vi "Peak Detector (obs 2010).vi"(4 "end of data (T)":bool=TRUE, 6 "initialize (T)":bool=TRUE, 8 "peaks/valleys":enum32{"Peaks", "Valleys"}(ring), 9 "width":i32=3 min=3, 10 "threshold":dbl format="%0.2f", 11 "X":dbl[](array[numeric])) -> (0 "error":i32, 1 "2nd Derivatives":dbl[](array[numeric]), 2 "Amplitudes":dbl[](array[numeric]), 3 "Locations":dbl[](array[numeric]), 5 "# found":i32)   [LabVIEW 2017, in "NI_AALPro.lvlib"]
doc: "Finds the location, amplitude, and second derivative of peaks or valleys in the input signal."
uses:
  NI_AALPro.lvlib
  <resource>/lvanlys.dll
panel:
  # "This VI is obsolete !\nYou should replace this VI in your digram with the Peak Detector VI."
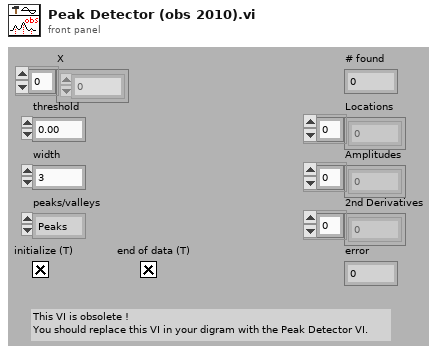
[diagram p1: front panel]
types:
  T1 = cluster{"Span":i32, "Index":i32, "NHistoryPts":i32, "Len":i32, "PrevSign":i32, "unused":i32, "RinvQt (pointer)":u32, "FitBuffer (pointer)":u32, "History (pointer)":u32, "PrevCoeff (pointer)":u32, "Data (pointer)":u32, "slack for RinvQt":u32, "slack for FitBuffer":u32, "slack for History":u32, "slack for PrevCoeff":u32, "slack for Data":u32}
  T2 = cluster{"X":dbl[], "threshold":dbl, "Span":i32, "peaks/valleys":enum32{"Peaks", "Valleys"}, "Array Constant":dbl[], "Array Constant":dbl[], "Array Constant":dbl[], i32, i32}
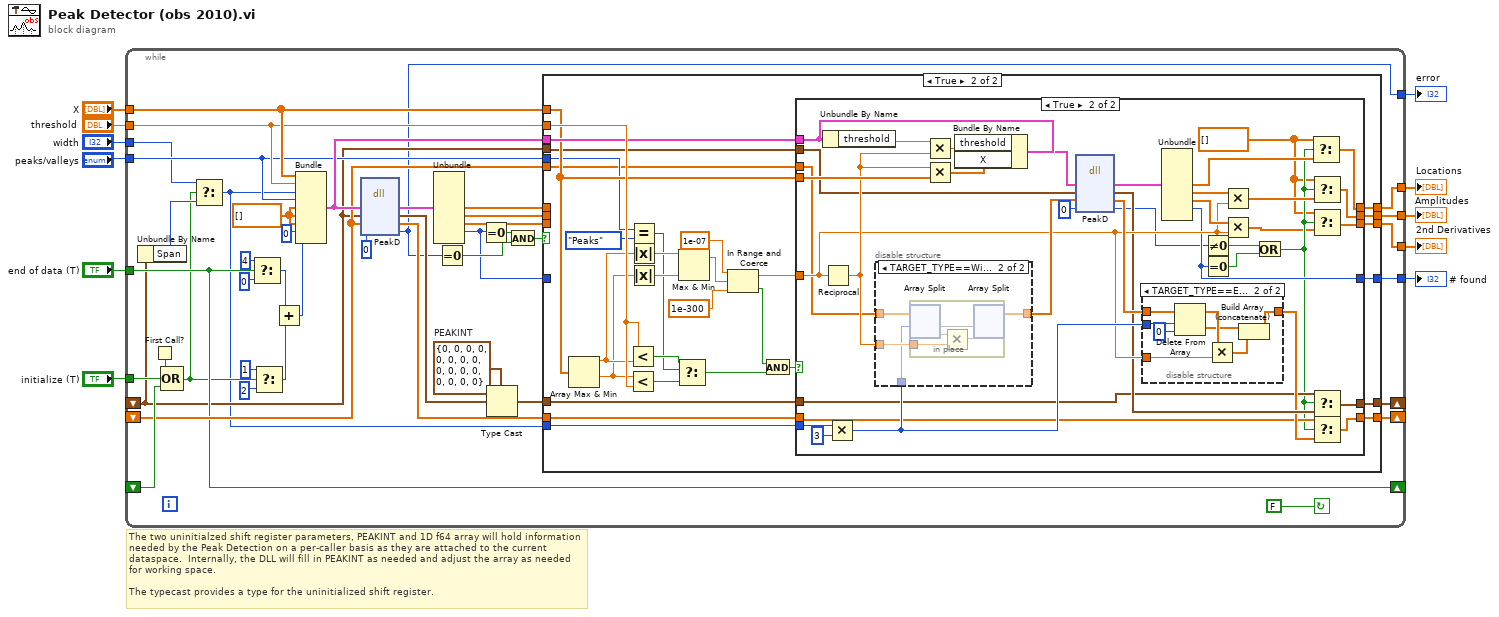
[diagram p0: block diagram]
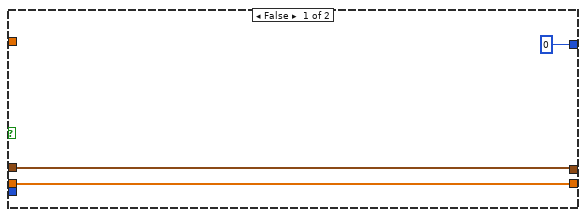
[diagram p3: hidden frame]
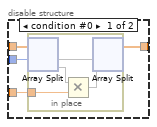
[diagram p4: hidden frame]
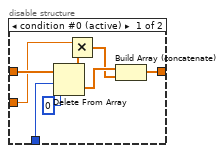
[diagram p5: hidden frame]
diagram:
  # "The two uninitialzed shift register parameters, PEAKINT and 1D f64 array will hold information needed by the Peak Detection on a per-caller basis as they are attached to the current dataspace.  Internally, the DLL will fill in PEAKINT as needed and adjust the array as needed for working space.\n\nThe typecast provides a type for the uninitialized shift register."
  n1 = while {
    shift-left: _ -> [w31]
    shift-right: [w33] -> _
    shift-left: _ -> [w17]
    shift-right: [w35] -> _
    shift-right: [w27] -> _
    shift-left: _ -> [w41]
    tunnel: "X" -> [w30]
    tunnel: "threshold" -> [w29]
    tunnel: "width" -> [w13]
    tunnel: "peaks/valleys" -> [w28]
    tunnel: "end of data (T)" -> [w27]
    tunnel: "initialize (T)" -> [w26]
    tunnel: [w12] -> w5
    tunnel: [w25] -> w4
    tunnel: [w24] -> w3
    tunnel: [w23] -> w2
    tunnel: [w22] -> w1
    stop <- FALSE continue-if-true
    w42 = T1 {"Span"=0, "Index"=0, "NHistoryPts"=0, "Len"=0, "PrevSign"=0, "unused"=0, "RinvQt (pointer)"=0, "FitBuffer (pointer)"=0, "History (pointer)"=0, "PrevCoeff (pointer)"=0, "Data (pointer)"=0, "slack for RinvQt"=0, "slack for FitBuffer"=0, "slack for History"=0, "slack for PrevCoeff"=0, "slack for Data"=0}  # PEAKINT
    w45 = dbl[] [] ("Array Constant")
    n2 = Unbundle By Name(w17) -> ("Span"=w16:i32)
    n3 = First Call?() -> (First Call?: T/F=w40:bool)
    n4 = Compound Arithmetic op=OR(w40, w26, w41) -> (w15:bool)
    n5 = Select(t=w13, s=w15, f=w16) -> (s? t:f=w14:i32)
    n6 = Select(t=4, s=w27, f=0) -> (s? t:f=w54:i32)
    n7 = Select(t=1, s=w15, f=2) -> (s? t:f=w55:i32)
    n8 = Add(x=w54, y=w55) -> (x+y=w48:i32)
    n9 = Bundle("X"=w30, "threshold"=w29, "Span"=w14, "peaks/valleys"=w28, "Array Constant"=w45, "Array Constant"=w45, "Array Constant"=w45, 0, w48) -> (w32:T2)  [unwired: 1 out]
    n10 = dll-call lib="C:/Program Files (x86)/National Instruments/LabVIEW 2017/resource/lvanlys.*" fn="PeakD"("PeakApp"=w32, "pPEAKINT"=w17, "SavedData"=w31, "pErr"=0) -> ("PeakApp"=w47:T2, "pPEAKINT"=w43:T1, "SavedData"=w34:dbl[], "pErr"=w12:i32)  [unwired: 3 in, 3 out]
    n11 = Unbundle(w47) -> ("Array Constant"=w37:dbl[], "Array Constant"=w38:dbl[], "Array Constant"=w39:dbl[], w18:i32)  [unwired: 5 out]
    n12 = Equal To 0?(x=w12) -> (x = 0?=w20:bool)
    n13 = Equal To 0?(x=w18) -> (x = 0?=w21:bool)
    n14 = Type Cast(type=w42, x=w43) -> (*(type *) &x=w36:T1)
    n15 = And(x=w21, y=w20) -> (x .and. y?=w19:bool)
    n16 = case shown="True" w19 {
      tunnel: w39 -> [w59 _]
      tunnel: w38 -> [w60 _]
      tunnel: w37 -> [w61 _]
      tunnel: w30 -> [_ w72]
      tunnel: w29 -> [_ w91]
      tunnel: w28 -> [_ w69]
      tunnel: w34 -> [w57 w80]
      tunnel: w36 -> [w58 w62]
      tunnel: [w58 w79] -> w35
      tunnel: [w57 w78] -> w33
      tunnel: [w59 w77] -> w23
      tunnel: [w60 w76] -> w24
      tunnel: [w61 w75] -> w25
      tunnel: w32 -> [_ w73]
      tunnel: w17 -> [_ w71]
      tunnel: w31 -> [_ w68]
      tunnel: [w56 w67] -> w22
      tunnel: w18 -> [w56 _]
      tunnel: w14 -> [_ w63]
      frame False {
      }
      frame True {
        n17 = Array Max & Min(array=w72) -> (max value=w88:dbl, min value=w87:dbl)  [unwired: 2 out]
        n18 = Less?(x=w91, y=w88) -> (x < y?=w90:bool)
        n19 = Less?(x=w87, y=w91) -> (x < y?=w89:bool)
        n20 = Equal?(x=w69, y=enum32{"Peaks", "Valleys"}."Peaks") -> (x = y?=w66:bool)
        n21 = Absolute Value(x=w88) -> (abs(x)=w86:dbl)
        n22 = Absolute Value(x=w87) -> (abs(x)=w85:dbl)
        n23 = Select(t=w90, s=w66, f=w89) -> (s? t:f=w84:bool)
        n24 = Max & Min(x=w86, y=w85) -> (max(x,y)=w82:dbl)  [unwired: 1 out]
        n25 = In Range and Coerce(upper limit=1e-07 ("y"), x=w82, lower limit=1e-300 ("y")) -> (coerced(x)=w74:dbl, In Range?=w81:bool)
        n26 = And(x=w81, y=w84) -> (x .and. y?=w83:bool)
        n27 = case shown="True" w83 {
          tunnel: w62 -> [w94 w110]
          tunnel: w80 -> [w93 w108]
          tunnel: [w94 w115] -> w79
          tunnel: [w93 w111] -> w78
          tunnel: [_ w100] -> w77
          tunnel: [_ w101] -> w76
          tunnel: [_ w103] -> w75
          tunnel: w74 -> [_ w118]
          tunnel: w73 -> [_ w130]
          tunnel: w72 -> [_ w129]
          tunnel: w71 -> [_ w114]
          tunnel: w68 -> [_ w112]
          tunnel: [0 w117] -> w67
          tunnel: w63 -> [_ w106]
          frame False {
          }
          frame True {
            w98 = dbl[] [] ("t")
            n28 = Unbundle By Name(w130) -> ("threshold"=w131:dbl)
            n29 = Reciprocal(x=w118) -> (1/x=w122:dbl)
            n30 = Multiply(x=w106, y=3) -> (x*y=w119:i32)
            n31 = disable-structure shown="TARGET_TYPE==Windows||TARGET_TYPE==Unix||TARGET_TYPE==Mac" {
              disable-tunnel: w122 -> [w151 w159]
              disable-tunnel: [w148 w158] -> w121
              disable-tunnel: w119 -> [w154 w157]
              disable-tunnel: w112 -> [w155 w156]
              frame condition #0 (active) {
                n32 = Delete From Array(array=w155, length=w154, index=0) -> (deleted portion=w150:dbl[], array with subset deleted=w152:dbl[])
                n33 = Multiply(x=w151, y=w152) -> (x*y=w149:dbl[])
                n34 = Build Array (concatenate)(w150, w149) -> (w148:dbl[])
              }
              frame condition #1 {
                n35 = in-place {
                  in-place-border: w159 -> [w161]
                  n36 = in-place-split #1(w156, w157) -> (w162:dbl[], w163:dbl[])
                  n37 = Multiply(x=w163, y=w161) -> (x*y=w160:dbl[])
                  n38 = in-place-split #1(w162, w160) -> (w158:dbl[])  [unwired: 1 out]
                }
              }
            }
            n39 = Multiply(x=w131, y=w122) -> (x*y=w128:dbl)
            n40 = Multiply(x=w122, y=w129) -> (x*y=w127:dbl[])
            n41 = Bundle By Name(cluster=w130, "threshold"=w128, "X"=w127) -> (w107:T2)
            n42 = dll-call lib="C:/Program Files (x86)/National Instruments/LabVIEW 2017/resource/lvanlys.*" fn="PeakD"("PeakApp"=w107, "pPEAKINT"=w114, "SavedData"=w121, "pErr"=0) -> ("PeakApp"=w125:T2, "pPEAKINT"=w116:T1, "SavedData"=w120:dbl[], "pErr"=w105:i32)  [unwired: 3 in, 3 out]
            n43 = disable-structure shown="TARGET_TYPE==Embedded||TARGET_TYPE==PocketPC, Default" {
              disable-tunnel: w120 -> [w135 w147]
              disable-tunnel: w119 -> [w134 w146]
              disable-tunnel: w118 -> [w133 w143]
              disable-tunnel: [w132 w140] -> w113
              frame condition #0 {
                n44 = in-place {
                  in-place-border: w133 -> [w137]
                  n45 = in-place-split #2(w135, w134) -> (w138:dbl[], w139:dbl[])
                  n46 = Multiply(x=w139, y=w137) -> (x*y=w136:dbl[])
                  n47 = in-place-split #2(w138, w136) -> (w132:dbl[])  [unwired: 1 out]
                }
              }
              frame condition #1 (active) {
                n48 = Delete From Array(array=w147, length=w146, index=0) -> (deleted portion=w142:dbl[], array with subset deleted=w144:dbl[])
                n49 = Multiply(x=w144, y=w143) -> (x*y=w141:dbl[])
                n50 = Build Array (concatenate)(w142, w141) -> (w140:dbl[])
              }
            }
            n51 = Unbundle(w125) -> ("Array Constant"=w104:dbl[], "Array Constant"=w124:dbl[], "Array Constant"=w123:dbl[], w117:i32)  [unwired: 5 out]
            n52 = Not Equal To 0?(x=w105) -> (x != 0?=w96:bool)
            n53 = Equal To 0?(x=w117) -> (x = 0?=w95:bool)
            n54 = Multiply(x=w124, y=w118) -> (x*y=w102:dbl[])
            n55 = Multiply(x=w123, y=w118) -> (x*y=w97:dbl[])
            n56 = Or(x=w96, y=w95) -> (x .or. y?=w99:bool)
            n57 = Select(t=w98, s=w99, f=w104) -> (s? t:f=w103:dbl[])
            n58 = Select(t=w98, s=w99, f=w102) -> (s? t:f=w101:dbl[])
            n59 = Select(t=w98, s=w99, f=w97) -> (s? t:f=w100:dbl[])
            n60 = Select(t=w110, s=w99, f=w116) -> (s? t:f=w115:T1)
            n61 = Select(t=w108, s=w99, f=w113) -> (s? t:f=w111:dbl[])
          }
        }
      }
    }
  }
  "Locations" <- w4
  "Amplitudes" <- w3
  "2nd Derivatives" <- w2
  "error" <- w5
  "# found" <- w1
